vi "To Array.vi"(4 "TypeMap":refnum<class "TypeMap.lvclass">, 7 "Type":refnum<class>, 8 "error in (no error)":errorcluster, 10 "Query Result in":refnum<class "Query Result.lvclass">, 11 "SqlMapper in":refnum<class "SqlMapper.lvclass">) -> (0 "error out":errorcluster, 2 "Array":refnum<class>[](array[class]), 3 "SqlMapper out":refnum<class "SqlMapper.lvclass">)   [LabVIEW 2020, in "ORM_API.lvlib"]
uses:
  ORM_API.lvlib
  <vilib>/Viviota/shared/ORM.lvlibp/ORM/Query Result/Query Result.lvclass
  <vilib>/Viviota/shared/ORM.lvlibp/ORM/SqlMapper/SqlMapper.lvclass
  <vilib>/Viviota/shared/ORM.lvlibp/ORM/TypeMap/TypeMap.lvclass
  <userlib>/_OpenG.lib/lvdata/lvdata.llb/LVOOP Is Default Value__ogtk.vi
  <vilib>/Viviota/shared/ORM.lvlibp/ORM/TypeMap/Read TypeMap.vi
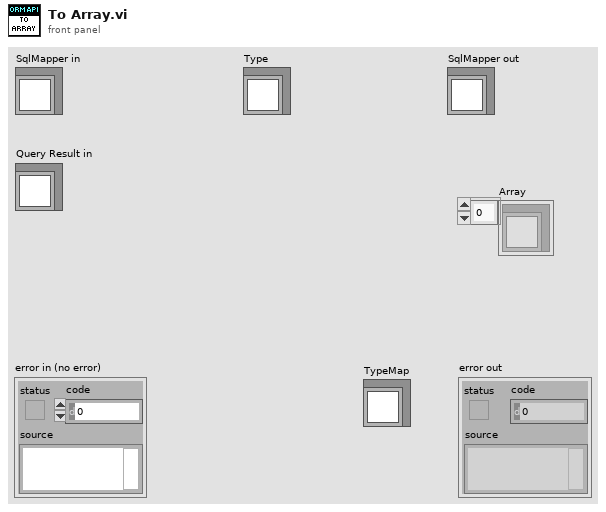
[diagram p1: front panel]
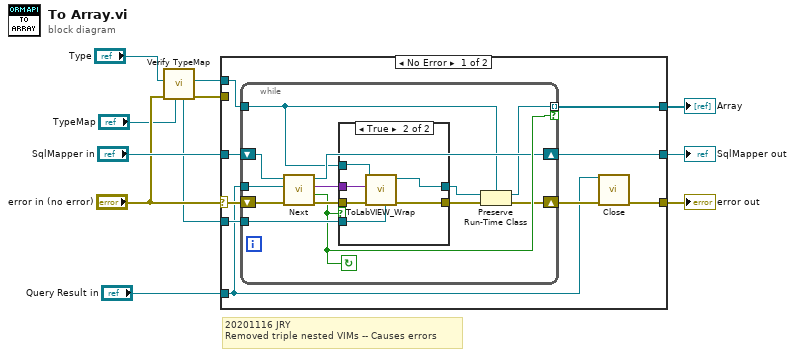
[diagram p0: block diagram]
diagram:
  # "20201116 JRY\nRemoved triple nested VIMs -- Causes errors"
  n1 = call "Verify TypeMap.vi"("TypeMap in"="TypeMap", "error in (no error)"="error in (no error)", "Type in"="Type") -> ("error out"=w1:errorcluster, "Type out"=w5:refnum<class>, "TypeMap out"=w3:refnum<class "TypeMap.lvclass">)  [unwired: 6 in]
  n2 = case shown="No Error" "error in (no error)" {
    selector: "error in (no error)" -> [w20 w43]
    tunnel: [w13 w43] -> w11
    tunnel: "Query Result in" -> [w12 _]
    tunnel: w5 -> [w18 _]
    tunnel: [w15 w42] -> w9
    tunnel: "SqlMapper in" -> [w17 w42]
    tunnel: w3 -> [w16 _]
    tunnel: [w14 _] -> w7
    tunnel: w1 -> [_ _]
    frame No Error {
      n3 = while {
        shift-right: [w24] -> w19
        shift-left: w20 -> [w31]
        tunnel: w18 -> [w21]
        tunnel: w16 -> [w29]
        shift-right: [w25] -> w15
        shift-left: w17 -> [w30]
        tunnel: w12 -> [w27]
        tunnel: [w22] -> w14 mode=indexing if=w26
        stop <- w26 continue-if-true
        n4 = call <vilib>:"Next.vi"("error in (no error)"=w31, "Query in"=w27, "SqlMapper in"=w30) -> ("error out"=w32:errorcluster, "found?"=w26:bool, "Row"=w33:variant, "SqlMapper out"=w25:refnum<class "SqlMapper.lvclass">)  [unwired: 5 in]
        n5 = case shown="True" w26 {
          tunnel: w21 -> [w35 w36]
          tunnel: w33 -> [_ w38]
          tunnel: [w35 w37] -> w23
          tunnel: w32 -> [w34 w40]
          tunnel: [w34 w39] -> w28
          tunnel: w29 -> [_ w41]
          frame False {
          }
          frame True {
            n6 = call <vilib>:"ToLabVIEW_Wrap.vi"("TypeMap in"=w41, "error in (no error)"=w40, "DbRow"=w38, "TargetObject In"=w36) -> ("error out"=w39:errorcluster, "Object Out"=w37:refnum<class>)  [unwired: 6 in]
          }
        }
        n7 = Preserve Run-Time Class(object in=w23, error in=w28, 2:w21) -> (object out=w22:refnum<class>, error out=w24:errorcluster)
      }
      n8 = call-dynamic "Close.vi"("error in (no error)"=w19, "Query Result in"=w12) -> ("error out"=w13:errorcluster)  [unwired: 9 in]
    }
    frame Error {
    }
  }
  "error out" <- w11
  "Array" <- w7
  "SqlMapper out" <- w9
